vi "PeakOf1D.vi"(5 "Restrict range":bool=TRUE, 7 "Method":enum16{"Max", "Gauss", "Gaussoffset", "Parabel"}(ring), 11 "Waveform Graph":i16[](graph)=[500, 512, 499, 532, 513, 534, 571, 585, 572, 598, 625, 661, 629, 660, 701, 669, 731, 702, 736, 720, 718, 727, 716, 657, 642, 620, 617, 599, 604, 599]) -> (2 "Index":dbl, 3 "Peak":dbl)   [LabVIEW 2011]
uses:
  <vilib>/Analysis/6fits.llb/Curve Fitting Criteria.ctl
  <vilib>/Analysis/NI_AALPro.lvlib
panel:
  out "width":dbl
  out "offset":dbl
  # "gauss fittet sch..."
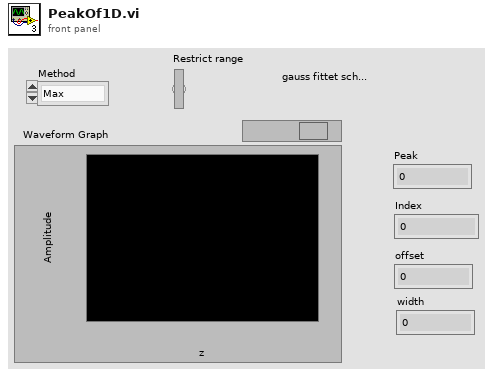
[diagram p1: front panel]
types:
  T1 = cluster{"initial amplitude":dbl, "initial center":dbl, "initial standard deviation":dbl, "offset":dbl}
  T2 = cluster{"amp min":dbl, "amp max":dbl, "center min":dbl, "center max":dbl, "deviation min":dbl, "deviation max":dbl, "offset min":dbl, "offset max":dbl}
  T3 = typedef "NI_AALPro.lvlib/Curve Fitting Criteria.ctl" = u16
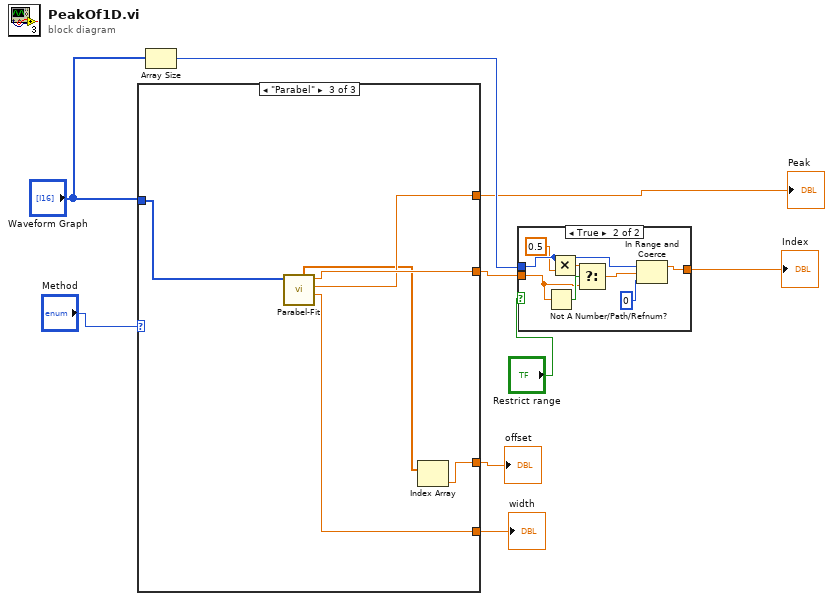
[diagram p0: block diagram]
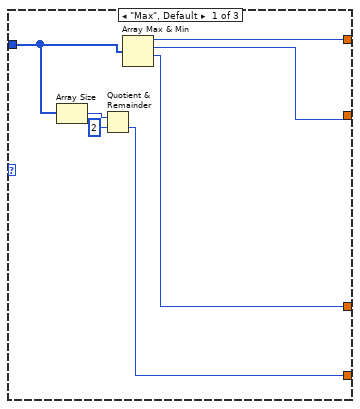
[diagram p3: hidden frame]
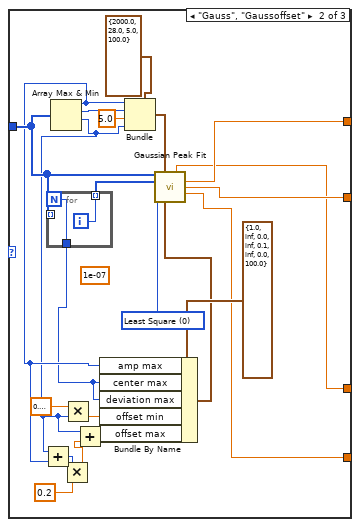
[diagram p4: hidden frame]
diagram:
  n1 = case shown="\"Parabel\"" "Method" {
    tunnel: "Waveform Graph" -> [w13 w34 w46]
    tunnel: [w16 w37 w44] -> w4
    tunnel: [w15 w38 w45] -> w7
    tunnel: [w14 w19 w41] -> w2
    tunnel: [w10 w17 w43] -> w1
    frame "Max", Default {
      n2 = Array Size(array=w13) -> (size(s)=w12:i32)
      n3 = Quotient & Remainder(x=w12, y=2) -> (floor(x/y)=w10:i32)  [unwired: 1 out]
      n4 = Array Max & Min(array=w13) -> (max value=w16:i16, max index (indices)=w15:i32, min value=w14:i16)  [unwired: 1 out]
    }
    frame "Gauss", "Gaussoffset" {
      (unwired) 1e-07 ("tolerance")
      w35 = T3 0 items=["Least Square", "Least Absolute Residual", "Bisquare"] ("method")
      n5 = for {
        N -> [w39]
        tunnel: w34 -> [_] mode=indexing
        tunnel: [w40] -> w36 mode=indexing
        tunnel: [w39] -> w25
        i -> [w40]
      }
      n6 = Array Max & Min(array=w34) -> (max value=w28:i16, max index (indices)=w32:i32, min value=w24:i16)  [unwired: 1 out]
      n7 = Add(x=w24, y=w28) -> (x+y=w27:i16)
      n8 = Multiply(x=w27, y=0.2) -> (x*y=w22:dbl)
      n9 = Multiply(x=sgl 0.8, y=w24) -> (x*y=w21:sgl)
      n10 = Add(x=w24, y=w22) -> (x+y=w23:dbl)
      n11 = Bundle By Name(cluster=T2 {"amp min"=1.0, "amp max"=inf, "center min"=0.0, "center max"=inf, "deviation min"=0.1, "deviation max"=inf, "offset min"=0.0, "offset max"=100.0} ("parameter bounds"), "amp max"=w28, "center max"=w25, "deviation max"=w25, "offset min"=w21, "offset max"=w23) -> (w29:T2)
      n12 = Bundle(cluster=T1 {"initial amplitude"=2000.0, "initial center"=28.0, "initial standard deviation"=5.0, "offset"=100.0} ("initial guess"), "initial amplitude"=w28, "initial center"=w32, "initial standard deviation"=5.0, "offset"=w24) -> (w33:T1)
      n13 = call <vilib>:"Gaussian Peak Fit.vi"("Y"=w34, "initial guess"=w33, "X"=w36, "method"=w35, "parameter bounds"=w29) -> ("offset"=w19:dbl, "amplitude"=w37:dbl, "center"=w38:dbl, "standard deviation"=w17:dbl)  [unwired: 4 in, 3 out]
    }
    frame "Parabel" {
      n14 = call "Parabel-Fit.vi"("data"=w46) -> ("FWHM"=w43:dbl, "Peek"=w44:dbl, "Position"=w45:dbl, "fit"=w42:dbl[])  [unwired: 7 in]
      n15 = Index Array(array=w42) -> (element=w41:dbl)  [unwired: 1 in]
    }
  }
  "Peak" <- w4
  "offset" <- w2
  "width" <- w1
  n16 = Array Size(array="Waveform Graph") -> (size(s)=w6:i32)
  n17 = case shown="True" "Restrict range" {
    tunnel: w7 -> [w47 w51]
    tunnel: w6 -> [_ w50]
    tunnel: [w47 w54] -> w5
    frame False {
    }
    frame True {
      n18 = Not A Number/Path/Refnum?(number/path/refnum=w51) -> (NaN/Path/Refnum?=w53:bool)
      n19 = Multiply(x=w50, y=0.5) -> (x*y=w49:dbl)
      n20 = Select(t=w49, s=w53, f=w51) -> (s? t:f=w52:dbl)
      n21 = In Range and Coerce(upper limit=w50, x=w52, lower limit=0) -> (coerced(x)=w54:dbl)  [unwired: 1 out]
    }
  }
  "Index" <- w5
